vi "SM Request Transition.vi"(7 "Req. Transition":refnum<user-event>, 8 "error in (no error)":errorcluster, 10 "Data":variant, 11 "Transition":T1) -> (0 "error out":errorcluster)   [LabVIEW 2020, in "StateMachine.lvlib" / "HSE-State-Machine.lvlib"]
doc: "Sends a Transition to the State Machine which will react dependent on it's state.\n____\nHAMPEL SOFTWARE ENGINEERING v2.6.0 (2023-12-19 10:54)"
uses:
  HSE-State-Machine.lvlib
  SM_Transitions.ctl
  SM Request Transition Argument--cluster.ctl
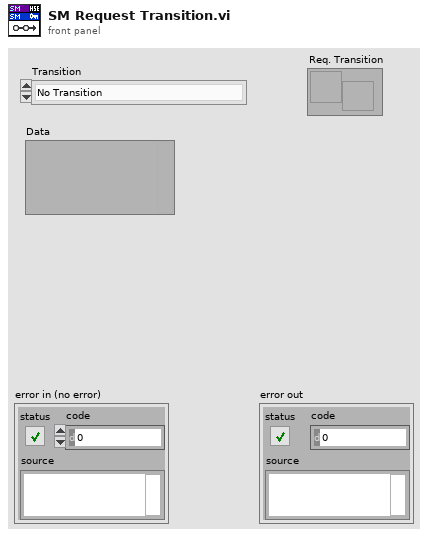
[diagram p1: front panel]
types:
  T1 = typedef "StateMachine.lvlib/HSE-State-Machine.lvlib/SM_Transitions.ctl" = enum16{"No Transition", "Exception", "Reset", "Initialization finished", "Process started", "Trigger detected", "Exit"}
  T2 = typedef "StateMachine.lvlib/HSE-State-Machine.lvlib/SM Request Transition Argument--cluster.ctl" = cluster{"Transition":T1, "Data":variant}
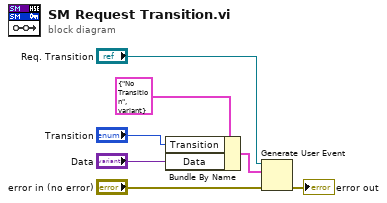
[diagram p0: block diagram]
diagram:
  n1 = Bundle By Name(cluster=T2 {"Transition"=enum."No Transition", "Data"=variant} ("Trigger HSE-SM Transition Argument"), "Transition"="Transition", "Data"="Data") -> (w6:T2)
  n2 = Generate User Event(user event="Req. Transition", event data cluster=w6, error in="error in (no error)") -> (error out=→"error out":errorcluster)  [unwired: 1 in, 1 out]
